vi "scanWaveGen_deBullshitFP.vi"(6 "overScanBlanking":bool, 8 "singleDirScan":bool, 9 "numRoundingPts":u16, 10 "scanWaveForm":T2, 11 "numPts":u16) -> (2 "blankingParams":T1, 3 "outWave":dbl[](array[numeric]))   [LabVIEW 2016]
uses:
  controls/ScanWaveform.ctl
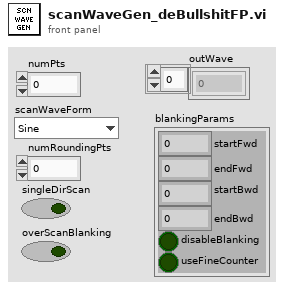
[diagram p1: front panel]
types:
  T1 = cluster{"startFwd":u16, "endFwd":u16, "startBwd":u16, "endBwd":u16, "disableBlanking":bool, "useFineCounter":bool}
  T2 = typedef "ScanWaveform.ctl" = enum16{"Sine", "Triangle", "Rounded"}
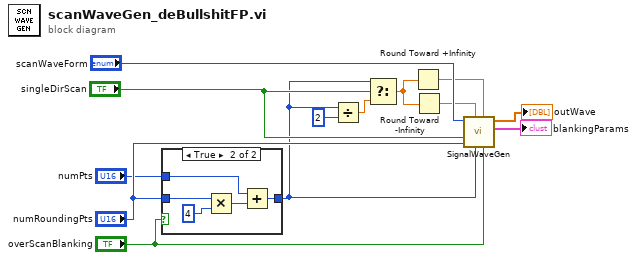
[diagram p0: block diagram]
diagram:
  n1 = case shown="True" "overScanBlanking" {
    tunnel: "numRoundingPts" -> [_ w19]
    tunnel: [w14 w16] -> w2
    tunnel: "numPts" -> [w14 w15]
    frame False {
    }
    frame True {
      n2 = Multiply(x=w19, y=u16 4) -> (x*y=w17:u16)
      n3 = Add(x=w15, y=w17) -> (x+y=w16:u16)
    }
  }
  n4 = Divide(x=w2, y=i16 2) -> (x/y=w7:dbl)
  n5 = Select(t=w2, s="singleDirScan", f=w7) -> (s? t:f=w8:dbl)
  n6 = Round Toward +Infinity(x=w8) -> (ceil(x): smallest int >= x=w4:dbl)
  n7 = Round Toward -Infinity(1:w8) -> (0:w3:dbl)
  n8 = call "SignalWaveGen.vi"("overScanBlanking"="overScanBlanking", "Numeric 2"=w4, "numPts"=w2, "Numeric"=w3, "numRoundingPts"="numRoundingPts", "singleDirScan"="singleDirScan", "scanWaveForm"="scanWaveForm") -> ("fastBlanking"=→"blankingParams":T1, "Array"=→"outWave":dbl[])  [unwired: 3 in]
